vi "NumericFactory.vi"(8 "error in":errorcluster, 11 "Gen Refnum":refnum<vi>) -> (0 "error out":errorcluster, 3 "Numeric out":refnum<class "Numeric.lvclass">)   [LabVIEW 2014, in "Numeric.lvclass"]
uses:
  Numeric.lvclass
  Digital/Digital.lvclass
  NamedNumeric/NamedNumeric.lvclass
  NumericWithScale/NumericWithScale.lvclass
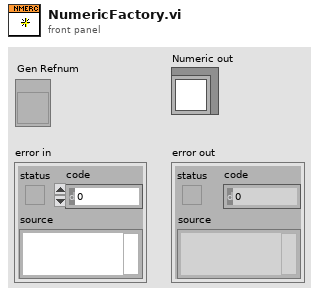
[diagram p1: front panel]
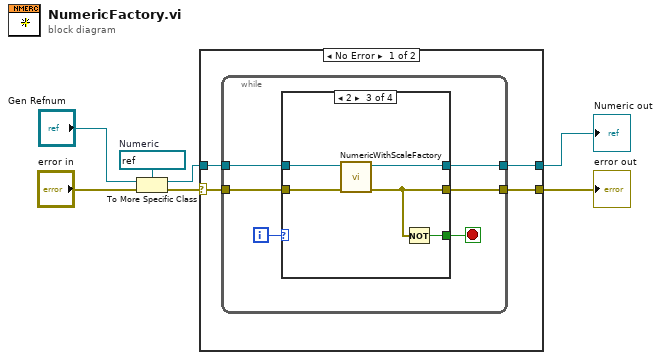
[diagram p0: block diagram]
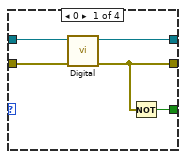
[diagram p2: hidden frame]
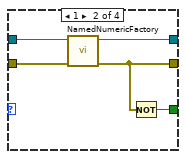
[diagram p3: hidden frame]
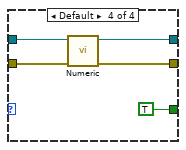
[diagram p4: hidden frame]
diagram:
  w5 = refnum<vi> refnum  # Numeric
  n1 = To More Specific Class(target class=w5, reference="Gen Refnum", error in="error in") -> (specific class reference=w3:refnum<vi>, error out=w4:errorcluster)
  n2 = case shown="No Error" w4 {
    selector: w4 -> [w11 w38]
    tunnel: [w9 _] -> w1
    tunnel: [w8 w38] -> w2
    tunnel: w3 -> [w10 _]
    frame No Error {
      n3 = while {
        tunnel: w11 -> [w16]
        tunnel: [w15] -> w8
        tunnel: [w14] -> w9
        tunnel: w10 -> [w12]
        i -> [w17]
        stop <- w13 stop-if-true
        n4 = case shown="2" w17 {
          tunnel: w16 -> [w22 w27 w32 w35]
          tunnel: [w19 w24 w29 w33] -> w15
          tunnel: [w21 w26 w31 w34] -> w14
          tunnel: [w20 w25 w30 TRUE] -> w13
          tunnel: w12 -> [w18 w23 w28 w36]
          frame 0 {
            n5 = call "Digital.vi"("error in"=w22, "GObj Refnum"=w18) -> ("error out"=w19:errorcluster, "Digital out"=w21:refnum<class "Digital.lvclass">)  [unwired: 8 in]
            n6 = Not(x=w19) -> (.not. x?=w20:bool)
          }
          frame 1 {
            n7 = call "NamedNumericFactory.vi"("error in"=w27, "Gen Refnum"=w23) -> ("error out"=w24:errorcluster, "NamedNumeric out"=w26:refnum<class "NamedNumeric.lvclass">)  [unwired: 8 in]
            n8 = Not(x=w24) -> (.not. x?=w25:bool)
          }
          frame 2 {
            n9 = call "NumericWithScaleFactory.vi"("error in"=w32, "Gen Refnum"=w28) -> ("error out"=w29:errorcluster, "NumericWithScale out"=w31:refnum<class "NumericWithScale.lvclass">)  [unwired: 8 in]
            n10 = Not(x=w29) -> (.not. x?=w30:bool)
          }
          frame Default {
            n11 = call "Numeric.vi"("error in"=w35, "GObj Refnum"=w36) -> ("error out"=w33:errorcluster, "Numeric out"=w34:refnum<class "Numeric.lvclass">)  [unwired: 8 in]
          }
        }
      }
    }
    frame Error {
    }
  }
  "error out" <- w2
  "Numeric out" <- w1
